vi "Get Plugged Channels.vi"(8 "error in (no error)":errorcluster, 11 "Potentiostat Galvanostat in":refnum<class "Potentiostat Galvanostat.lvclass">) -> (0 "error out":errorcluster, 1 "Plugged Channels":u8[](array[ring]) items=["Channel 0", "Channel 1", "Channel 2", "Channel 3", "Channel 4", "Channel 5", "Channel 6", "Channel 7", "Channel 8", "Channel 9", "Channel 10", "Channel 11", "Channel 12", "Channel 13", "Channel 14", "Channel 15"], 3 "Potentiostat Galvanostat out":refnum<class "Potentiostat Galvanostat.lvclass">)   [LabVIEW 2018, in "Potentiostat Galvanostat.lvclass"]
uses:
  Potentiostat Galvanostat.lvclass
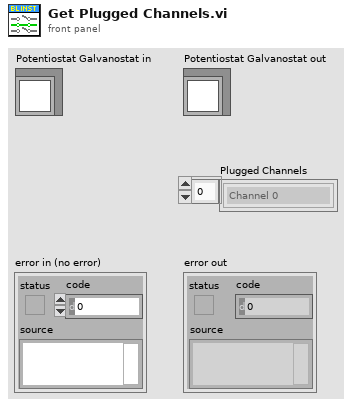
[diagram p1: front panel]
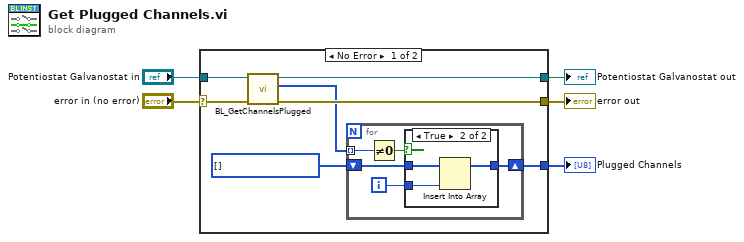
[diagram p0: block diagram]
diagram:
  n1 = case shown="No Error" "error in (no error)" {
    selector: "error in (no error)" -> [w9 w23]
    tunnel: [w8 w23] -> w4
    tunnel: [w10 w22] -> w2
    tunnel: "Potentiostat Galvanostat in" -> [w12 w22]
    tunnel: [w6 _] -> w1
    frame No Error {
      w11 = u8[] [] items=["Channel 0", "Channel 1", "Channel 2", "Channel 3", "Channel 4", "Channel 5", "Channel 6", "Channel 7", "Channel 8", "Channel 9", "Channel 10", "Channel 11", "Channel 12", "Channel 13", "Channel 14", "Channel 15"]
      n2 = call-dynamic "BL_GetChannelsPlugged .vi"("error in (no error)"=w9, "Potentiostat Galvanostat in"=w12) -> ("error out"=w8:errorcluster, "Plugged Channels"=w7:u8[], "Potentiostat Galvanostat out"=w10:refnum<class "Potentiostat Galvanostat.lvclass">)  [unwired: 7 in]
      n3 = for {
        tunnel: w7 -> [w16] mode=indexing
        shift-right: [w13] -> w6
        shift-left: w11 -> [w17]
        i -> [w14]
        n4 = Not Equal To 0?(x=w16) -> (x != 0?=w15:bool)
        n5 = case shown="True" w15 {
          tunnel: w17 -> [w18 w21]
          tunnel: w14 -> [_ w20]
          tunnel: [w18 w19] -> w13
          frame False {
          }
          frame True {
            n6 = Insert Into Array(array=w21, new element=w20) -> (w19:u8[])  [unwired: 1 in]
          }
        }
      }
    }
    frame Error {
    }
  }
  "error out" <- w4
  "Potentiostat Galvanostat out" <- w2
  "Plugged Channels" <- w1
